vi "onDeserializeParameters.vi"(8 "error in (no error)":errorcluster, 10 "Variant":variant, 11 "RequirementMap in":refnum<class "TraceabilityMatrix.lvclass">) -> (0 "error out":errorcluster, 3 "RequirementMap out":refnum<class "TraceabilityMatrix.lvclass">)   [LabVIEW 2021, in "Bananas.lvlib" / "TraceabilityMatrix.lvclass"]
uses:
  TraceabilityMatrix.lvclass
  params -- cluster.ctl
  TraceabilityMatrix.lvclass/TraceabilityMatrix.ctl
  <vilib>/LabVIEW Open Source Project/Data Manipulation/TypeDescriptor/TypeDescriptor_GetType.vi
  <vilib>/LabVIEW Open Source Project/Data Manipulation/TypeDescriptor/TypeDescriptor_GetName.vi
  <vilib>/LabVIEW Open Source Project/Data Manipulation/Variant/Variant_EmptyCluster.vi
  <vilib>/LabVIEW Open Source Project/Data Manipulation/TypeDescriptor/TypeDescriptor_GetPString.vi
  <vilib>/Utility/GetType.llb/Get Type Code from I16 Array And Pos.vi
  <vilib>/Utility/GetType.llb/TD_Create Cluster.vi
  BananaPeel/BananaPeel.lvclass
  <vilib>/LabVIEW Open Source Project/Data Manipulation/Variant/OpenVariant.lvlib
  <vilib>/LabVIEW Open Source Project/OpenURI/uri/URI.lvclass
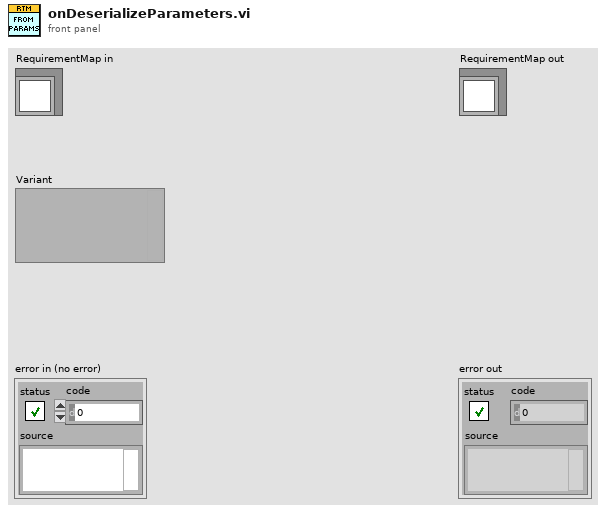
[diagram p1: front panel]
types:
  T1 = typedef "Type Enum.ctl" = enum8{"Void", "I8", "I16", "I32", "I64", "U8", "U16", "U32", "U64", "Single Float", "Double Float", "Extended Float", "Single Complex", "Double Complex", "Extended Complex", "Enum I8 NEVER", "Enum I16 NEVER", "Enum I32 NEVER", "Enum I64 NEVER", "Enum U8", "Enum U16", "Enum U32", "Enum U64", "Single Float With Unit", "Double Float With Unit", "Extended Float With Unit", "Single Complex With Unit", "Double Complex With Unit", "Extended Complex With Unit", "boolU16", "Boolean", "String", "Handle", "Path", "Picture", "C String", "Pascal String", "Tag", "SubString", "Array", "SubArray", "Cluster", "Numeric Cluster", "Variant", "LV Variant", "Measure Data (waveform)", "Refnum", "ExtData", "function", "Typedef", "Poly VI", "bad wire", "LabVIEW Class Instance"}
  T2 = typedef "Bananas.lvlib/TraceabilityMatrix.lvclass/params -- cluster.ctl" = cluster{"uri":string, "type":string, "start-row":string, "start-col":string}
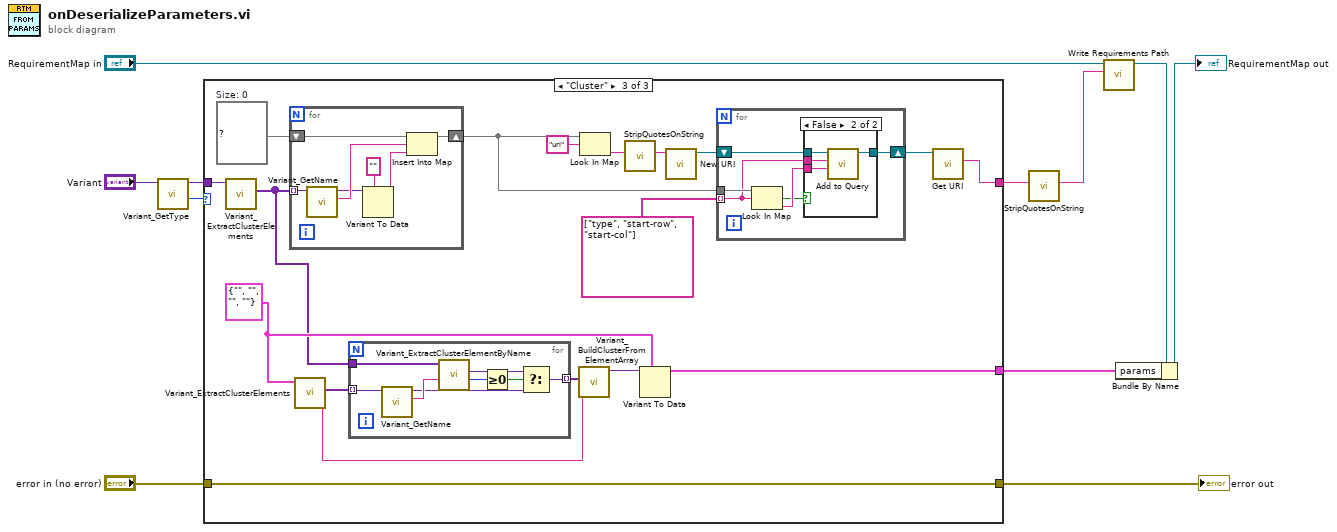
[diagram p0: block diagram]
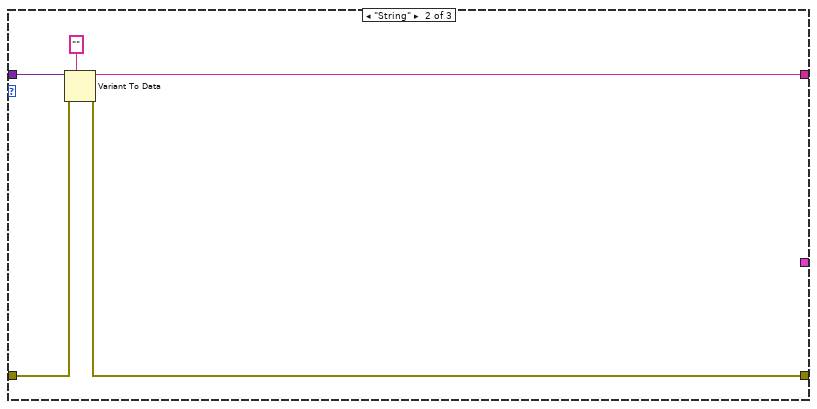
[diagram p3: hidden frame]
diagram:
  n1 = call <vilib>:"Variant_GetType.vi"("Variant"="Variant") -> ("Type Enum"=w6:T1, "Variant dup"=w4:variant)  [unwired: 8 in, 1 out]
  n2 = case shown="\"Cluster\"" w6 {
    tunnel: [_ w17 w33] -> w9
    tunnel: "error in (no error)" -> [w12 w16 w32]
    tunnel: [w12 w15 w32] -> w7
    tunnel: w4 -> [_ w13 w31]
    tunnel: [_ _ w18] -> w1
    frame Default {
    }
    frame "String" {
      n3 = Variant To Data(error in=w16, type="", Variant=w13) -> (data=w17:string, error out=w15:errorcluster)
    }
    frame "Cluster" {
      w20 = T2 {"uri"="", "type"="", "start-row"="", "start-col"=""} ("params")
      w30 = map{string, string} {}  # Size: 0
      n4 = call <vilib>:"Variant_ExtractClusterElements.vi"("Cluster"=w31) -> ("Elements"=w19:variant[])  [unwired: 8 in, 2 out]
      n5 = for {
        tunnel: w19 -> [w61] mode=indexing
        shift-right: [w59] -> w27
        shift-left: w30 -> [w58]
        n6 = call <vilib>:"Variant_GetName.vi"("Variant"=w61) -> ("Name"=w60:string, "Variant dup"=w56:variant)  [unwired: 8 in, 1 out]
        n7 = Variant To Data(type="" ("name"), Variant=w56) -> (data=w55:string)  [unwired: 1 in, 1 out]
        n8 = Insert Into Map(map in=w58, key=w60, value=w55) -> (map out=w59:map{string, string})  [unwired: 2 out]
      }
      n9 = call <vilib>:"Variant_ExtractClusterElements.vi"("Cluster"=w20) -> ("name"=w22:string, "Elements"=w24:variant[])  [unwired: 8 in, 1 out]
      n10 = for {
        tunnel: w24 -> [w43] mode=indexing
        tunnel: w19 -> [w42]
        tunnel: [w36] -> w23 mode=indexing
        n11 = call <vilib>:"Variant_GetName.vi"("Variant"=w43) -> ("Name"=w41:string, "Variant dup"=w37:variant)  [unwired: 8 in, 1 out]
        n12 = call <vilib>:"Variant_ExtractClusterElementByName.vi"("name"=w41, "Cluster"=w42) -> ("index"=w40:i32, "Element"=w38:variant)  [unwired: 7 in, 1 out]
        n13 = Greater Or Equal To 0?(x=w40) -> (x >= 0?=w39:bool)
        n14 = Select(t=w38, s=w39, f=w37) -> (s? t:f=w36:variant)
      }
      n15 = call <vilib>:"Variant_BuildClusterFromElementArray.vi"("name"=w22, "Elements"=w23) -> ("Cluster"=w21:variant)  [unwired: 9 in]
      n16 = Look In Map(map=w27, key="uri" ("name")) -> (value=w28:string)  [unwired: 1 in, 1 out]
      n17 = call "StripQuotesOnString.vi"("String"=w28) -> ("Unquoted String"=w35:string)  [unwired: 10 in]
      n18 = Variant To Data(type=w20, Variant=w21) -> (data=w18:T2)  [unwired: 1 in, 1 out]
      n19 = call <vilib>:"New URI.vi"("URI"=w35) -> ("URI"=w34:refnum<class "URI.lvclass">)  [unwired: 9 in, 1 out]
      n20 = for {
        tunnel: w27 -> [w48]
        tunnel: string[] ["type", "start-row", "start-col"] -> [w45] mode=indexing
        shift-right: [w44] -> w26
        shift-left: w34 -> [w49]
        n21 = Look In Map(map=w48, key=w45) -> (key not found?=w46:bool, value=w47:string)  [unwired: 1 in]
        n22 = case shown="False" w46 {
          tunnel: w49 -> [w50 w54]
          tunnel: [w50 w53] -> w44
          tunnel: w45 -> [_ w52]
          tunnel: w47 -> [_ w51]
          frame True {
          }
          frame False {
            n23 = call <vilib>:"Add to Query.vi"("value"=w51, "key"=w52, "URI in"=w54) -> ("URI out"=w53:refnum<class "URI.lvclass">)  [unwired: 7 in, 1 out]
          }
        }
      }
      n24 = call <vilib>:"Get URI.vi"("URI in"=w26) -> ("URI String"=w33:string)  [unwired: 8 in, 2 out]
    }
  }
  "error out" <- w7
  n25 = call "StripQuotesOnString.vi"("String"=w9) -> ("Unquoted String"=w11:string)  [unwired: 10 in]
  n26 = call "Write Requirements Path.vi"("URI"=w11, "Project in"="RequirementMap in") -> ("Project out"=w3:refnum<class "TraceabilityMatrix.lvclass">)  [unwired: 9 in]
  n27 = Bundle By Name(cluster=w3, "params"=w1) -> (→"RequirementMap out":refnum<class "TraceabilityMatrix.lvclass">)
